vi "Read AI Line.vi"(7 "AI line":T1=4000 items=["ModA/AI0"=4000, "ModA/AI1"=4001, "ModA/AI2"=4002, "ModA/AI3"=4003, "ModA/AI4"=4004, "ModA/AI5"=4005, "ModA/AI6"=4006, "ModA/AI7"=4007, "ModA/AI8"=4008, "ModA/AI9"=4009], 8 "error in (no error)":errorcluster, 11 "starter kit host in":refnum<class "NI_Robotics_Starter Kit Host.lvclass">) -> (0 "error out":errorcluster, 2 "data":dbl, 3 "starter kit host out":refnum<class "NI_Robotics_Starter Kit Host.lvclass">)   [LabVIEW 2017, in "NI_Robotics_Starter Kit Host.lvclass"]
doc: "Reads the voltage value from an analog input line on the Starter Kit FPGA."
uses:
  <vilib>/robotics/Starter Kit/Host Interface/NI_Robotics_Starter Kit Host.lvclass
  <vilib>/robotics/Starter Kit/Direct IO/AI Lines.ctl
  <vilib>/robotics/Starter Kit/Host Interface/NI_Robotics_Starter Kit Host.lvclass/NI_Robotics_Starter Kit Host.ctl
  <vilib>/robotics/Utilities/Generate Error.vi
  <vilib>/robotics/Starter Kit/Direct IO/NI_Robotics_Starter Kit Direct IO.lvclass
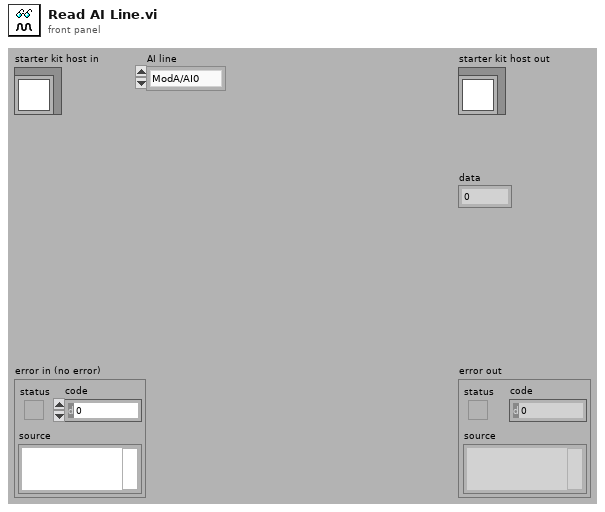
[diagram p1: front panel]
types:
  T1 = typedef "NI_Robotics_Starter Kit Direct IO.lvclass/AI Lines.ctl" = u16
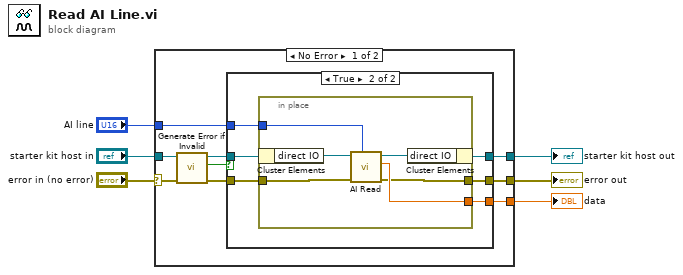
[diagram p0: block diagram]
diagram:
  n1 = case shown="No Error" "error in (no error)" {
    selector: "error in (no error)" -> [w9 w31]
    tunnel: [w13 w31] -> w2
    tunnel: [w15 w30] -> w3
    tunnel: "starter kit host in" -> [w11 w30]
    tunnel: "AI line" -> [w14 _]
    tunnel: [w12 _] -> w1
    frame No Error {
      n2 = call <vilib>:"Generate Error if Invalid.vi"("error in (no error)"=w9, "starter kit host in"=w11) -> ("error out"=w8:errorcluster, "valid?"=w7:bool, "starter kit host out"=w10:refnum<class "NI_Robotics_Starter Kit Host.lvclass">)  [unwired: 7 in]
      n3 = case shown="True" w7 {
        tunnel: [w17 w23] -> w15
        tunnel: w14 -> [_ w22]
        tunnel: [w16 w21] -> w13
        tunnel: [_ w20] -> w12
        tunnel: w10 -> [w17 w19]
        tunnel: w8 -> [w16 w18]
        frame False {
        }
        frame True {
          n4 = in-place {
            in-place-border: w18 -> [w25]
            in-place-border: [w26] -> w21
            in-place-border: w22 -> [w24]
            in-place-border: [w27] -> w20
            n5 = in-place-cluster #1(w19) -> ("direct IO"=w29:refnum<class "NI_Robotics_Starter Kit Direct IO.lvclass">)
            n6 = call-dynamic "AI Read.vi"("AI line"=w24, "error in (no error)"=w25, "direct IO in"=w29) -> ("error out"=w26:errorcluster, "data"=w27:dbl, "direct IO out"=w28:refnum<class "NI_Robotics_Starter Kit Direct IO.lvclass">)  [unwired: 6 in]
            n7 = in-place-cluster #1("direct IO"=w28) -> (w23:refnum<class "NI_Robotics_Starter Kit Host.lvclass">)
          }
        }
      }
    }
    frame Error {
    }
  }
  "error out" <- w2
  "starter kit host out" <- w3
  "data" <- w1
